vi "New JSON Null.vi"(8 "error in (no error)":errorcluster) -> (0 "error out":errorcluster, 3 "JSON Null out":refnum<class "JSON Helper.lvclass">)   [LabVIEW 2016, in "JSON Helper.lvclass"]
doc: "Create a new JSON instance with no assigned value"
uses:
  JSON Helper/JSON Helper.lvclass
  JSON Null.lvclass
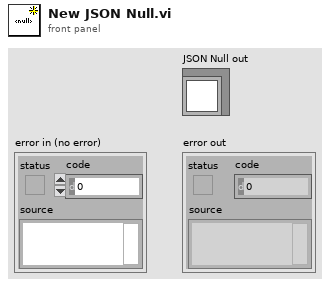
[diagram p1: front panel]
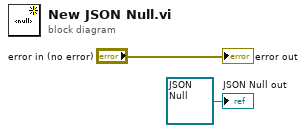
[diagram p0: block diagram]
diagram:
  "error out" <- "error in (no error)"
  "JSON Null out" <- refnum<class "JSON Null.lvclass"> refnum ("JSON String out")
